vi "Update Status Bar Cycles TEST.vi"(4 "Instrument String":i32, 5 "StatusBar":refnum<k7>) -> (1 "dup StatusBar":refnum<k7>)   [LabVIEW 2011]
panel:
  in  "StatusBar 2":refnum<k7>
  out "error out":errorcluster
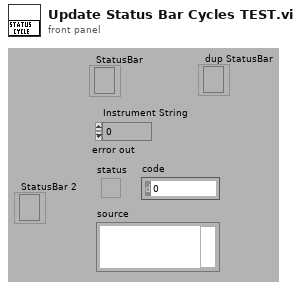
[diagram p1: front panel]
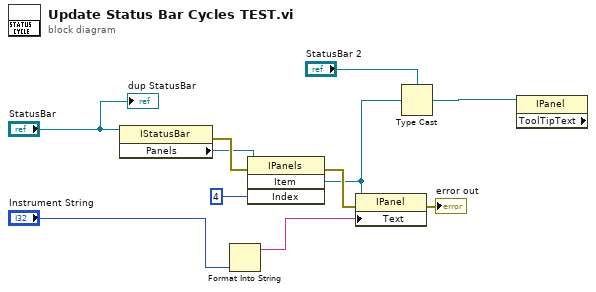
[diagram p0: block diagram]
diagram:
  n1 = property class="IStatusBar"(reference="StatusBar") -> (error out=w9:errorcluster, "Panels"=w4:refnum<k7>)  [unwired: 1 in, 1 out]
  n2 = Format Into String("Instrument String") -> (resulting string=w6:string)  [unwired: 3 in, 1 out]
  n3 = invoke class="IPanels" method="Item"(reference=w4, error in=w9, "Index"=4) -> (error out=w10:errorcluster, "Item"=w3:refnum<k7>)  [unwired: 1 in, 2 out]
  n4 = property class="IPanel"(reference=w3, error in=w10, "Text"=w6) -> (error out=→"error out":errorcluster)  [unwired: 1 out]
  n5 = Type Cast(type="StatusBar 2", x=w3) -> (*(type *) &x=w1:refnum<k7>)
  n6 = property class="IPanel" props=["ToolTipText"](reference=w1) -> ()  [unwired: 1 in, 3 out]
  "dup StatusBar" <- "StatusBar"
